vi "Get_LV_values_from_PS.vi"(8 "error in (no error)":errorcluster, 11 "Response":string) -> (0 "error out":errorcluster, 1 "Content":string, 2 "Headers":string, 3 "Status Description":string, 4 "Errors":string, 5 "Status Code":i32)   [LabVIEW 2016]
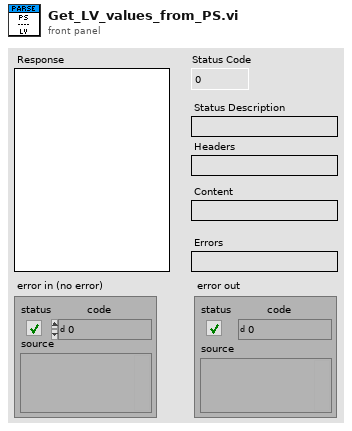
[diagram p1: front panel]
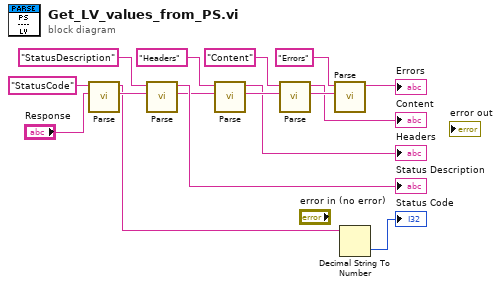
[diagram p0: block diagram]
diagram:
  n1 = call "Parse.vi"("String In"="Response", "RegEx"="StatusCode" ("regular expression")) -> ("After String"=w15:string, "Content"=w12:string)  [unwired: 8 in]
  n2 = call "Parse.vi"("String In"=w15, "RegEx"="StatusDescription" ("regular expression")) -> ("After String"=w4:string, "Content"=→"Status Description":string)  [unwired: 8 in]
  n3 = call "Parse.vi"("String In"=w4, "RegEx"="Headers" ("regular expression")) -> ("After String"=w9:string, "Content"=→"Headers":string)  [unwired: 8 in]
  n4 = call "Parse.vi"("String In"=w9, "RegEx"="Content") -> ("After String"=w6:string, "Content"=→"Content":string)  [unwired: 8 in]
  n5 = call "Parse.vi"("String In"=w6, "RegEx"="Errors") -> ("Content"=→"Errors":string)  [unwired: 8 in, 1 out]
  n6 = Decimal String To Number(string=w12) -> (number=→"Status Code":i32)  [unwired: 2 in, 1 out]
